vi "close.vi"(8 "error in (no error)":errorcluster, 11 "ZanCard in":refnum<class "ZanCard.lvclass">) -> (0 "error out":errorcluster, 3 "ZanCard out":refnum<class "ZanCard.lvclass">)   [LabVIEW 2019, in "ZanCard.lvclass"]
uses:
  ZanCard.lvclass
  ZanCard.lvclass/ZanCard.ctl
  LLB/zmotion/zaux/zauxdll.lvlib
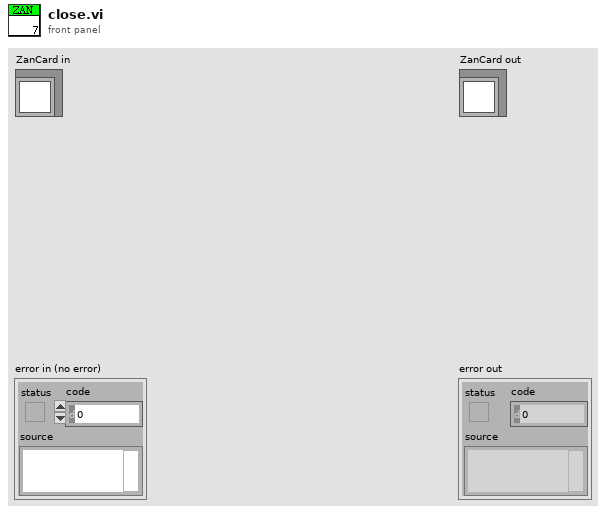
[diagram p1: front panel]
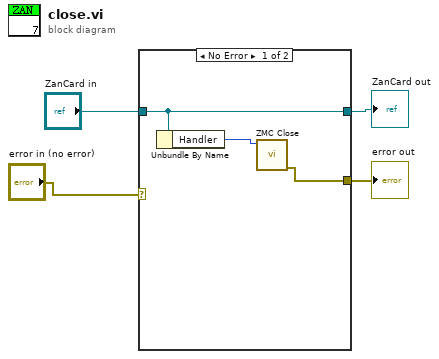
[diagram p0: block diagram]
diagram:
  n1 = case shown="No Error" "error in (no error)" {
    selector: "error in (no error)" -> [_ w8]
    tunnel: "ZanCard in" -> [w5 w9]
    tunnel: [w6 w8] -> w2
    tunnel: [w5 w9] -> w1
    frame No Error {
      n2 = Unbundle By Name(w5) -> ("Handler"=w7:i32)
      n3 = call "ZMC Close.vi"("handle"=w7) -> ("error out"=w6:errorcluster)  [unwired: 8 in, 2 out]
    }
    frame Error {
    }
  }
  "error out" <- w2
  "ZanCard out" <- w1
